vi "Var3.vi"() -> ()   [LabVIEW 2013]
panel:
  out "Ёмкость конденсатора, мкФ":dbl
  out "Величина заряда, мКл":dbl
  out "Сила тока":dbl(graph)
  out "Заряд":dbl(graph)
  out "Время разряда, сек":dbl
  in  "Uконечное, В":dbl
  out "Напряжение":dbl(graph)
  out "Напряжение конденсатора":dbl(knob) scale=0.1..10.0
  in  "Напряжение, В":dbl
  in  "Сопротивление, Ом":dbl
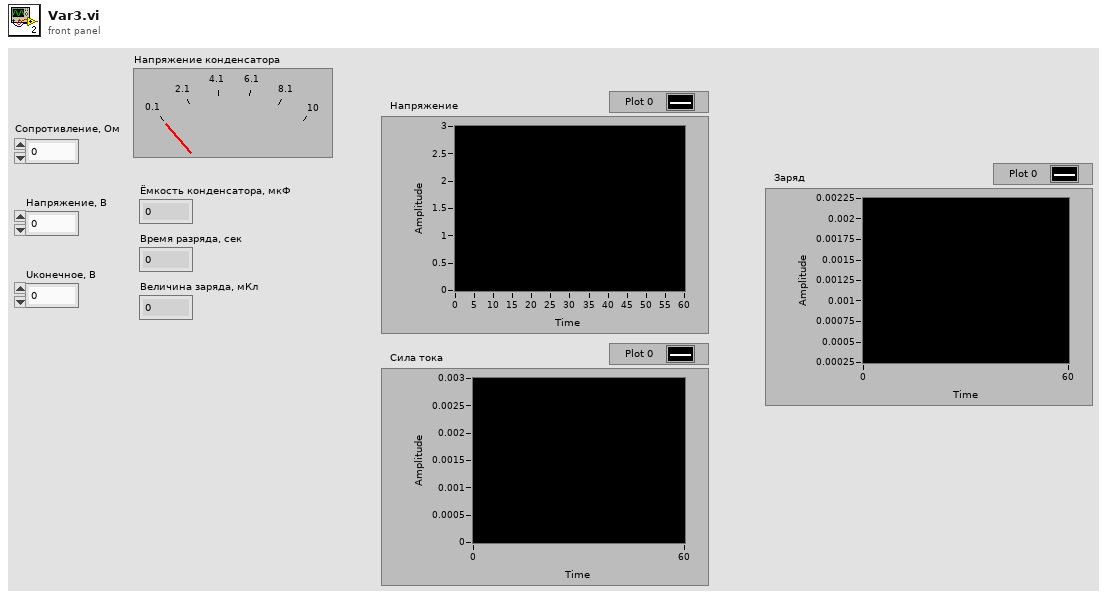
[diagram p1: front panel]
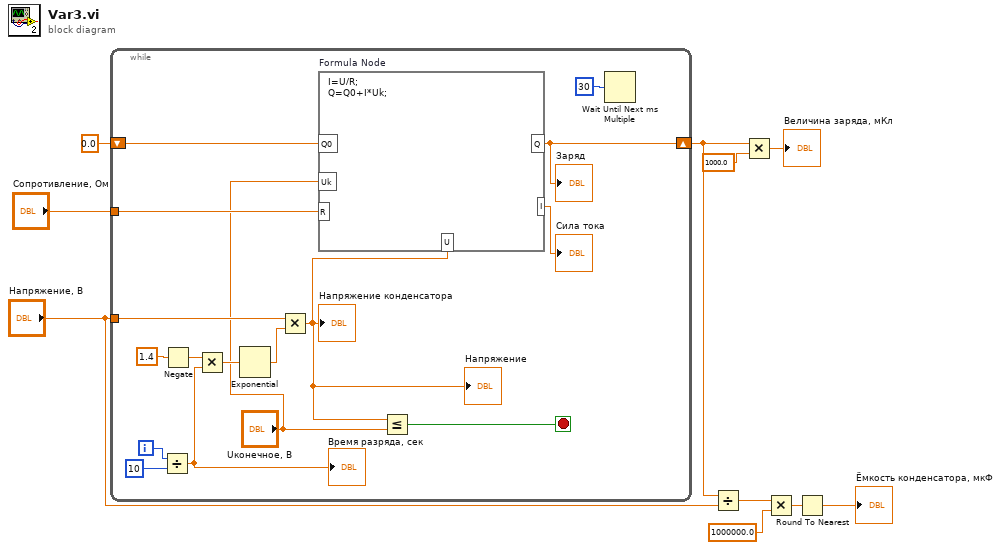
[diagram p0: block diagram]
diagram:
  n1 = while {
    shift-right: [w13] -> w6
    shift-left: 0.0 -> [w25]
    tunnel: "Сопротивление, Ом" -> [w24]
    tunnel: "Напряжение, В" -> [w18]
    i -> [w20]
    stop <- w16 stop-if-true
    n2 = Divide(x=w20, y=10) -> (x/y=w15:dbl)
    "Время разряда, сек" <- w15
    n3 = Negate(x=1.4) -> (-x=w22:dbl)
    n4 = Multiply(x=w22, y=w15) -> (x*y=w19:dbl)
    n5 = Exponential(1:w19) -> (0:w17:dbl)
    n6 = Multiply(x=w18, y=w17) -> (x*y=w11:dbl)
    "Напряжение конденсатора" <- w11
    "Напряжение" <- w11
    n7 = formula code="I=U/R;\nQ=Q0+I*Uk;"("Q0"=w25, "R"=w24, "U"=w11, "Uk"="Uконечное, В") -> ("I"=→"Сила тока":dbl, "Q"=w13:dbl)
    "Заряд" <- w13
    n8 = Less Or Equal?(x=w11, y="Uконечное, В") -> (x <= y?=w16:bool)
    n9 = Wait Until Next ms Multiple(millisecond multiple=u32 30 ("millisecond timer value")) -> ()  [unwired: 1 out]
  }
  n10 = Divide(x=w6, y="Напряжение, В") -> (x/y=w7:dbl)
  n11 = Multiply(x=w6, y=1000.0) -> (x*y=→"Величина заряда, мКл":dbl)
  n12 = Multiply(x=w7, y=1000000.0) -> (x*y=w2:dbl)
  n13 = Round To Nearest(number=w2) -> (nearest integer value=→"Ёмкость конденсатора, мкФ":dbl)
